vi "hipot ac test.vi"(8 "error in":errorcluster) -> (0 "error out":errorcluster)   [LabVIEW 2020]
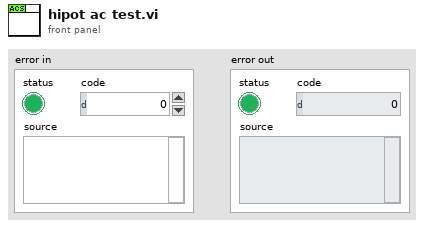
[diagram p1: front panel]
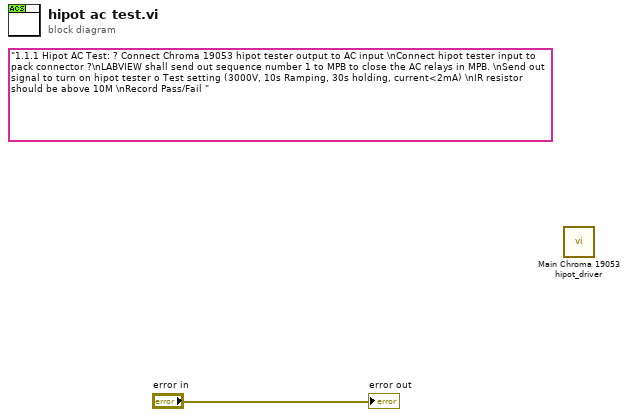
[diagram p0: block diagram]
diagram:
  (unwired) "1.1.1 Hipot AC Test: ? Connect Chroma 19053 hipot tester output to AC input \nConnect hipot tester input to pack connector ?\nLABVIEW shall send out sequence number 1 to MPB to close the AC relays in MPB. \nSend out signal to turn on hipot tester o Test setting (3000V, 10s Ramping, 30s holding, current<2mA) \nIR resistor should be above 10M \nRecord Pass/Fail "
  n1 = call "Main Chroma 19053 hipot_driver.vi"() -> ()  [unwired: 12 in]
  "error out" <- "error in"
